vi "Read Major and Minor Frames.vi"(8 "error in":errorcluster, 11 "port":T3 format="%.0x") -> (0 "error out":errorcluster, 1 "minor frames":T1[](array[typedef]), 2 "major frames":T2[](array[typedef]), 3 "port out":T3 format="%.0x")   [LabVIEW 2020, in "AIM MIL-STD-1553 Scripting.lvlib"]
doc: "Returns all <b>major frames</b> and <b>minor frames</b> within the <b>port</b>."
uses:
  AIM MIL-STD-1553 Scripting.lvlib
  <vilib>/NI VeriStand/Custom Device API/Custom Device Item Ref.ctl
  Shared/Major Frame Definition.ctl
  Shared/Minor Frame Definition.ctl
  Constants.vi
  <vilib>/NI VeriStand/Custom Device API/Get Item Property (String Array).vi
  <vilib>/NI VeriStand/Custom Device API/Custom Device API.lvlib
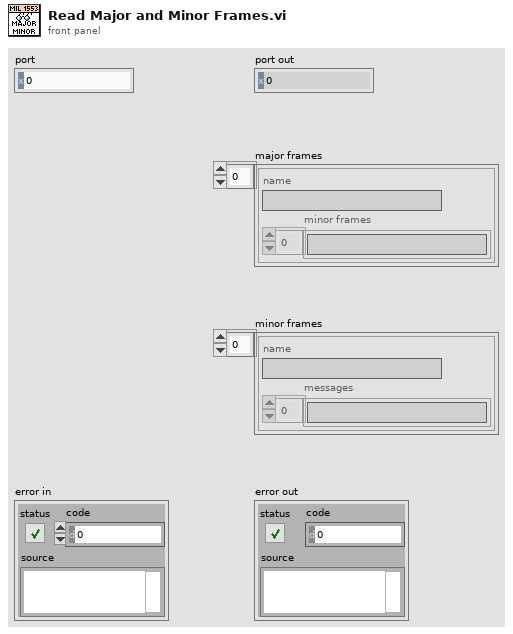
[diagram p1: front panel]
types:
  T1 = typedef "Minor Frame Definition.ctl" = cluster{"name":string, "messages":string[]}
  T2 = typedef "Major Frame Definition.ctl" = cluster{"name":string, "minor frames":string[]}
  T3 = typedef "Custom Device API.lvlib/Custom Device Item Ref.ctl" = u64
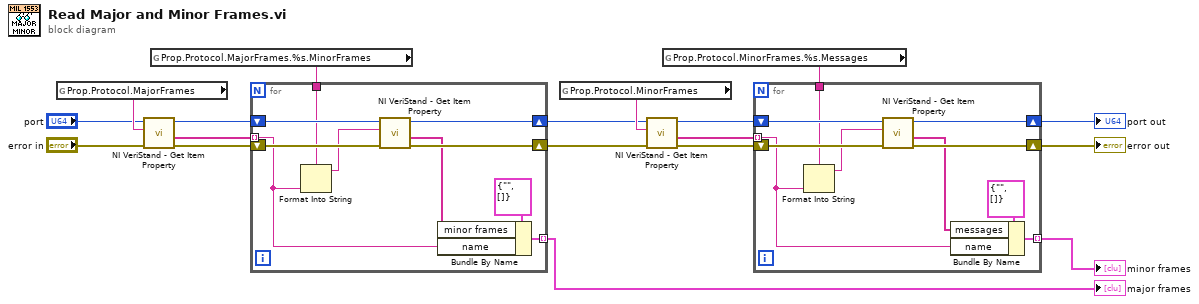
[diagram p0: block diagram]
diagram:
  n1 = global read "Constants.vi" "Prop.Protocol.MajorFrames"() -> (w9:string)
  n2 = call-poly <vilib>:"NI VeriStand - Get Item Property.vi"("error in (no error)"="error in", "Property Name"=w9, "Item Ref in"="port") -> ("error out"=w12:errorcluster, "Value"=w11:string[], "Item Ref out"=w10:T3)  [unwired: 5 in, 1 out]
  n3 = global read "Constants.vi" "Prop.Protocol.MajorFrames.%s.MinorFrames"() -> (w8:string)
  n4 = for {
    shift-right: [w26] -> w6
    shift-left: w12 -> [w25]
    shift-right: [w27] -> w5
    shift-left: w10 -> [w28]
    tunnel: w8 -> [w23]
    tunnel: w11 -> [w22] mode=indexing
    tunnel: [w20] -> w7 mode=indexing
    n5 = Format Into String(format string=w23, w22) -> (resulting string=w24:string)  [unwired: 2 in, 1 out]
    n6 = call-poly <vilib>:"NI VeriStand - Get Item Property.vi"("error in (no error)"=w25, "Property Name"=w24, "Item Ref in"=w28) -> ("error out"=w26:errorcluster, "Value"=w21:string[], "Item Ref out"=w27:T3)  [unwired: 5 in, 1 out]
    n7 = Bundle By Name(cluster=T2 {"name"="", "minor frames"=[]} ("major frame definition"), "minor frames"=w21, "name"=w22) -> (w20:T2)
  }
  "major frames" <- w7
  n8 = global read "Constants.vi" "Prop.Protocol.MinorFrames"() -> (w17:string)
  n9 = call-poly <vilib>:"NI VeriStand - Get Item Property.vi"("error in (no error)"=w6, "Property Name"=w17, "Item Ref in"=w5) -> ("error out"=w14:errorcluster, "Value"=w15:string[], "Item Ref out"=w16:T3)  [unwired: 5 in, 1 out]
  n10 = global read "Constants.vi" "Prop.Protocol.MinorFrames.%s.Messages"() -> (w18:string)
  n11 = for {
    shift-right: [w36] -> w1
    shift-left: w14 -> [w35]
    shift-right: [w37] -> w2
    shift-left: w16 -> [w38]
    tunnel: w18 -> [w33]
    tunnel: w15 -> [w32] mode=indexing
    tunnel: [w30] -> w13 mode=indexing
    n12 = Format Into String(format string=w33, w32) -> (resulting string=w34:string)  [unwired: 2 in, 1 out]
    n13 = call-poly <vilib>:"NI VeriStand - Get Item Property.vi"("error in (no error)"=w35, "Property Name"=w34, "Item Ref in"=w38) -> ("error out"=w36:errorcluster, "Value"=w31:string[], "Item Ref out"=w37:T3)  [unwired: 5 in, 1 out]
    n14 = Bundle By Name(cluster=T1 {"name"="", "messages"=[]} ("minor frame definition"), "messages"=w31, "name"=w32) -> (w30:T1)
  }
  "error out" <- w1
  "port out" <- w2
  "minor frames" <- w13
